vi "AO.vi"() -> ()   [LabVIEW 2016]
panel:
  out "error out":errorcluster caption="错误输出"
  in  "Voltage":sgl caption="DioOut"
  in  "DaNum":u8
  # "DaNum：DA通道号，0~3。如果设置为7，则表示为4个通道同时设置"
  # "Voltage：电压，0~10V"
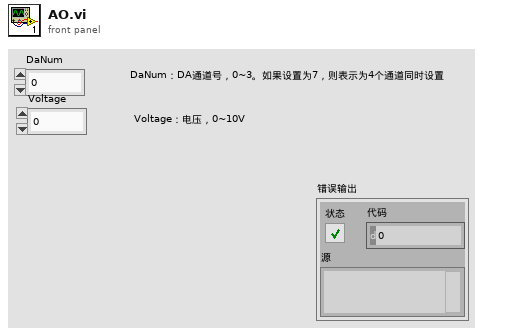
[diagram p1: front panel]
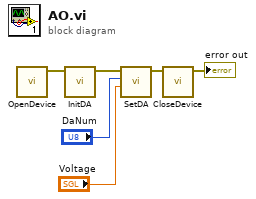
[diagram p0: block diagram]
diagram:
  n1 = call "OpenDevice.vi"() -> ("error out"=w6:errorcluster)  [unwired: 11 in]
  n2 = call "InitDA.vi"("error in"=w6) -> ("error out"=w5:errorcluster)  [unwired: 10 in]
  n3 = call "SetDA.vi"("Voltage"="Voltage", "DaNum"="DaNum", "error in"=w5) -> ("error out"=w4:errorcluster)  [unwired: 8 in]
  n4 = call "CloseDevice.vi"("error in"=w4) -> ("error out"=→"error out":errorcluster)  [unwired: 10 in]
